vi "Convert.vi"(8 "error in (no error)":errorcluster) -> (0 "error out":errorcluster)   [LabVIEW 2026]
panel:
  out "JSON out":string
  in  "VI Path in":path
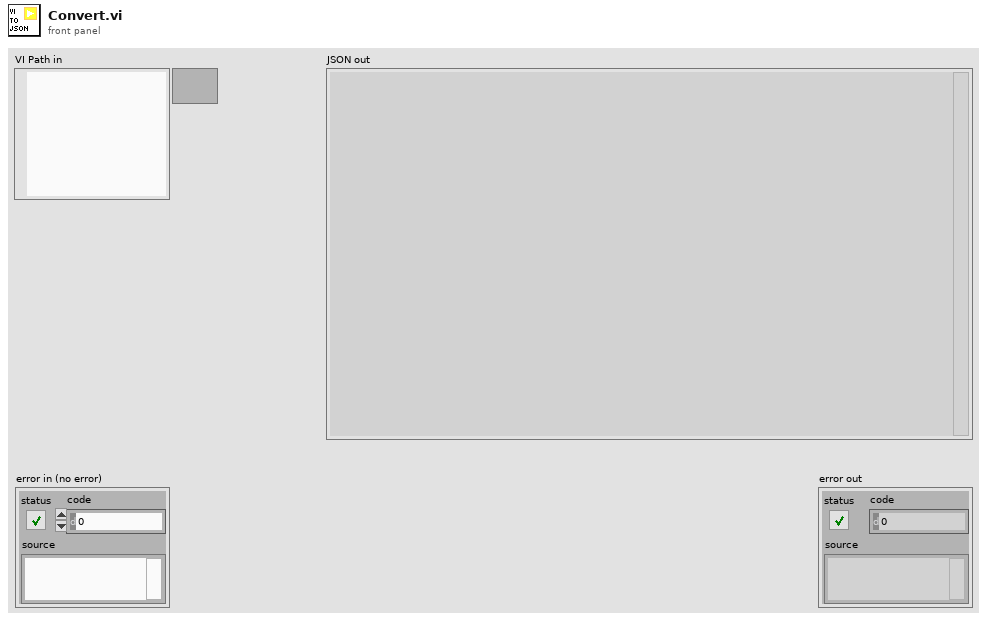
[diagram p1: front panel]
types:
  T1 = typedef "imagedata.ctl" = cluster{"image type":i32, "image depth":i32, "image":u8[], "mask":u8[], "colors":u32[], "Rectangle":cluster{"left":i16, "top":i16, "right":i16, "bottom":i16}}
  T2 = cluster{"Documentation/Icon":cluster{"Name":string, "Description":string, "ImageData":T1}, "Images":cluster{"Image":T1, "Child Indexes":i32[]}[]}
  T3 = typedef "JSON Image Data.ctl" = cluster{"Image":string, "Position":T4, "Children":dbl[]}
  T4 = typedef "Image Position.ctl" = cluster{"Left":i16, "Top":i16, "Width":i16, "Height":i16}
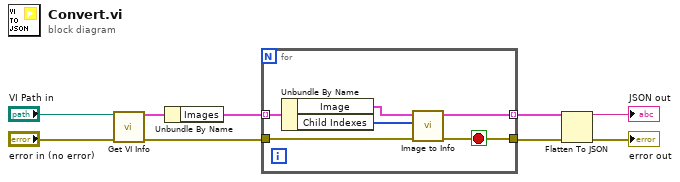
[diagram p0: block diagram]
diagram:
  n1 = call "Get VI Info.vi"("error in (no error)"="error in (no error)", "VI Path in"="VI Path in") -> ("error out"=w2:errorcluster, "VI Info out"=w8:T2)  [unwired: 8 in]
  n2 = Unbundle By Name(w8) -> ("Images"=w7:cluster{"Image":T1, "Child Indexes":i32[]}[])
  n3 = for {
    tunnel: w7 -> [w15] mode=indexing
    tunnel: [w11] -> w6 mode=indexing
    tunnel: w2 -> [w12]
    tunnel: [w10] -> w1
    stop <- w10 stop-if-true
    n4 = Unbundle By Name(w15) -> ("Image"=w14:T1, "Child Indexes"=w13:i32[])
    n5 = call "Image to Info.vi"("error in (no error)"=w12, "Child Indexes"=w13, "Image in"=w14) -> ("error out"=w10:errorcluster, "JSON Image out"=w11:T3)  [unwired: 7 in]
  }
  n6 = Flatten To JSON(anything=w6, error in (no error)=w1) -> (JSON string=→"JSON out":string, 11:→"error out":errorcluster)  [unwired: 1 in]
